vi "SCLN_GlobalStrings.vi"(2 "Write Value":string, 3 "Element":i32, 4 "Operation":i32 min=0 max=1, 5 "Number of Elements":i32=30) -> (0 "String Array Out":string[](array[string]), 1 "Read Value":string)   [LabVIEW 2015]
doc: "Handle String Globals Style II.\nThe globals are maintained in a\nshift register, as an array of String.\nTherefore, it is mandatory to initialize each element\nwith the first invocation wiring the\nnumber of elements to be contained in the array.\nThe elements will be initialized to vacio.\n\nINPUTS:\n Number of Elements : Use only on first\n call to initialize the array.\n Operation: 1 = WRITE, 0 = READ\n Element: Element of the array to write or read\n Write Value: String value to store\nOUTPUTS:\n Read Value: String value retrieved\n String Array Out: The entire array of Strings"
panel:
  # "1 = WRITE"
  # "0 = READ"
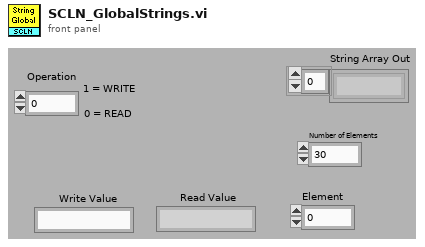
[diagram p1: front panel]
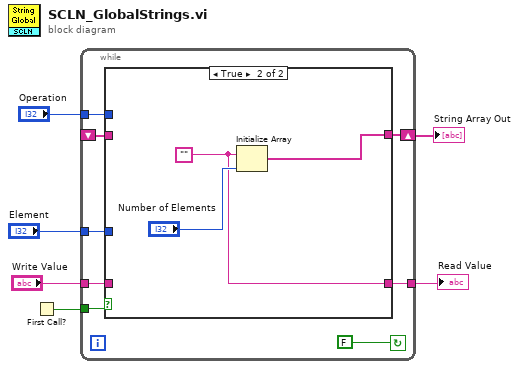
[diagram p0: block diagram]
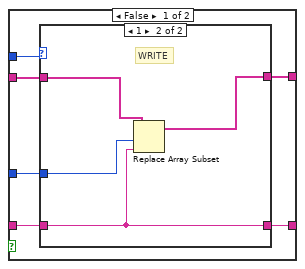
[diagram p2: hidden frame]
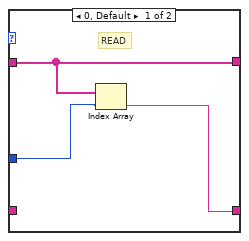
[diagram p3: hidden frame]
diagram:
  n1 = First Call?() -> (First Call?: T/F=w1:bool)
  n2 = while {
    shift-right: [w9] -> w2
    shift-left: _ -> [w8]
    tunnel: "Operation" -> [w13]
    tunnel: "Element" -> [w12]
    tunnel: "Write Value" -> [w11]
    tunnel: [w10] -> w3
    tunnel: w1 -> [w7]
    stop <- FALSE continue-if-true
    n3 = case shown="True" w7 {
      tunnel: w13 -> [w20 _]
      tunnel: w12 -> [w19 _]
      tunnel: w11 -> [w18 _]
      tunnel: [w17 w28] -> w10
      tunnel: [w16 w29] -> w9
      tunnel: w8 -> [w15 _]
      frame False {
        n4 = case shown="1" w20 {
          tunnel: w19 -> [w22 w27]
          tunnel: w18 -> [_ w26]
          tunnel: [w21 w26] -> w17
          tunnel: [w23 w25] -> w16
          tunnel: w15 -> [w23 w24]
          frame 0, Default {
            # "READ"
            n5 = Index Array(array=w23, index=w22) -> (element=w21:string)
          }
          frame 1 {
            # "WRITE"
            n6 = Replace Array Subset(array=w24, new element=w26, index=w27) -> (w25:string[])
          }
        }
      }
      frame True {
        w28 = ""
        n7 = Initialize Array(w28, "Number of Elements") -> (w29:string[])
      }
    }
  }
  "String Array Out" <- w2
  "Read Value" <- w3
